vi "Untitled 5.vi"   [LabVIEW 2020]
uses:
  24042b4b-bb26-41eb-832a-bdb45e894eeb.vi
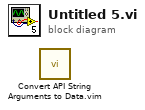
[diagram p0: block diagram]
diagram:
  n1 = call "Convert API String Arguments to Data.vim"() -> ()  [unwired: 8 in, 2 out]
